vi "smart invert.vi"() -> ()   [LabVIEW 2020]
uses:
  <vilib>/Analysis/coordinate.llb/Angle Units.ctl
  <vilib>/Analysis/coordinate.llb/Absolute Angle Difference (scalar).vi
  <vilib>/Analysis/coordinate.llb/Wrap Angle (scalar).vi
  <vilib>/Analysis/coordinate.llb/Set Angle Unit.vi
  <vilib>/Analysis/NI_AAL_Angle.lvlib
panel:
  out "absolute angle difference":dbl
  in  "Current Rotation Degrees":dbl
  out "Azimuth Setpoint":dbl
  out "Drive Out":dbl
  in  "Drive In":dbl
  in  "Desired Rotation Degrees":dbl
  # "encoder reads 990"
  # "requested rotation is 45 degrees"
  # "990 mod 360 = 2, remainder 270"
  # "45 degrees = 225 degrees"
  # "so we either want 720-45 or 720+225"
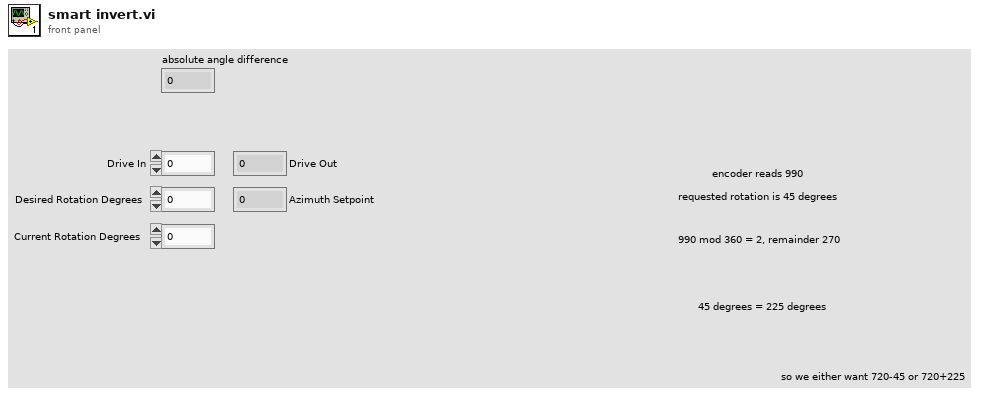
[diagram p1: front panel]
types:
  T1 = typedef "NI_AAL_Angle.lvlib/Angle Units.ctl" = i32
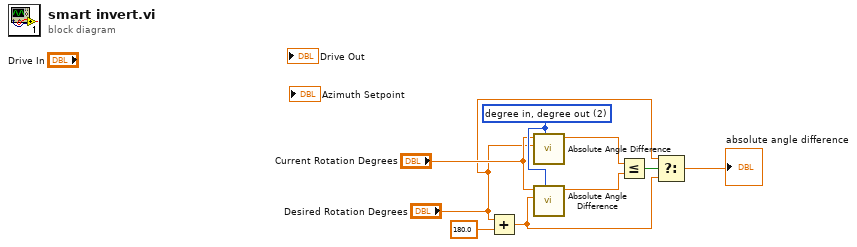
[diagram p0: block diagram]
diagram:
  w9 = T1 2 items=["radian in, radian out", "radian in, degree out", "degree in, degree out", "degree in, radian out"] ("angle units")
  n1 = Add(x="Desired Rotation Degrees", y=180.0) -> (x+y=w2:dbl)
  n2 = call-poly <vilib>:"Absolute Angle Difference.vi"("angle units"=w9, "angle 2"="Desired Rotation Degrees", "angle 1"="Current Rotation Degrees") -> ("absolute angle difference"=w6:dbl)  [unwired: 7 in, 1 out]
  n3 = call-poly <vilib>:"Absolute Angle Difference.vi"("angle units"=w9, "angle 2"=w2, "angle 1"="Current Rotation Degrees") -> ("absolute angle difference"=w5:dbl)  [unwired: 7 in, 1 out]
  n4 = Less Or Equal?(x=w6, y=w5) -> (x <= y?=w4:bool)
  n5 = Select(t="Desired Rotation Degrees", s=w4, f=w2) -> (s? t:f=→"absolute angle difference":dbl)
